vi "Message FGV.vi"(7 "Message Q FGV Actions":T2, 8 "error in":errorcluster) -> (0 "error out":errorcluster, 1 "remaining elements":T1[](array[typedef]), 2 "flushed elements":T1[](array[typedef]), 3 "queue ref out":refnum<queue>)   [LabVIEW 2020, in "Hardware.lvlib"]
doc: "Handle message queue reference operations for this component.\n\n<b>Create</b> - Obtain a message queue reference and store it in a Feedback Node.\n<b>Get</b> - Retrieve a previously stored message queue reference from the Feedback Node.\n<b>Destroy</b> - Destroy the stored message queue reference."
uses:
  Hardware.lvlib
  Message FGV Actions.ctl
  Message Type.ctl
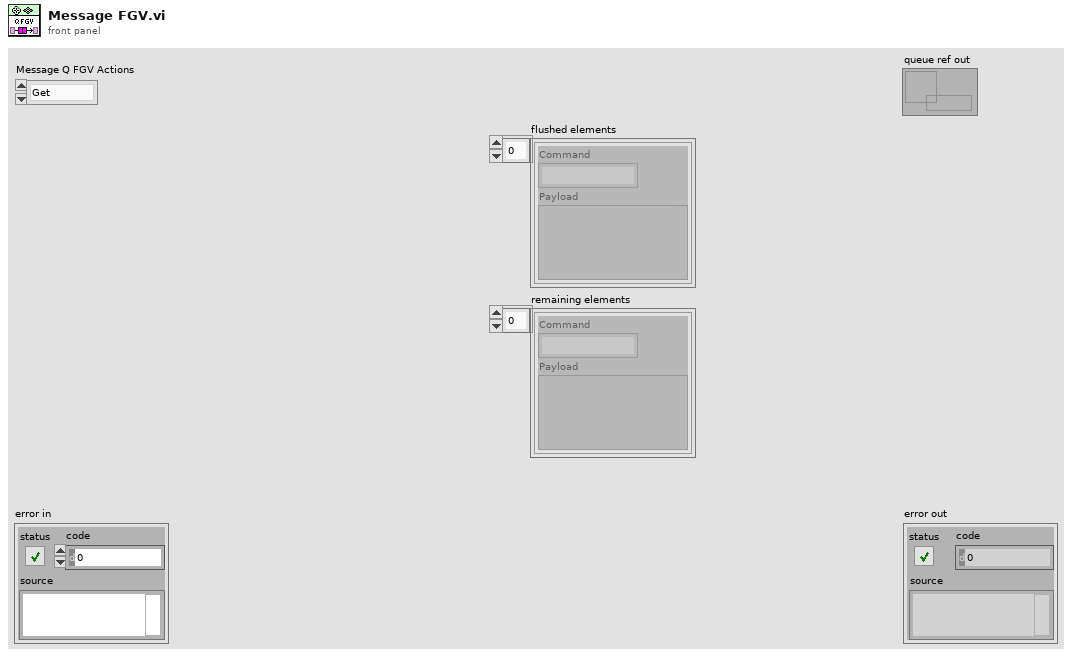
[diagram p1: front panel]
types:
  T1 = typedef "Hardware.lvlib/Message Type.ctl" = cluster{"Command":string, "Payload":variant}
  T2 = typedef "Hardware.lvlib/Message FGV Actions.ctl" = enum16{"Get", "Obtain", "Release", "Flush"}
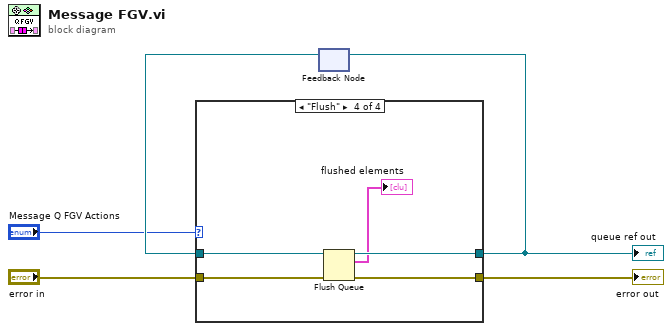
[diagram p0: block diagram]
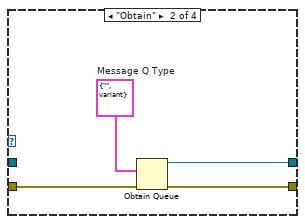
[diagram p3: hidden frame]
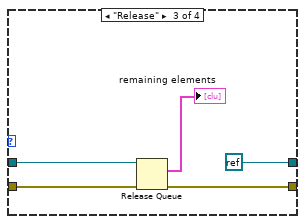
[diagram p4: hidden frame]
diagram:
  n1 = feedback #1() -> (w2:refnum<queue>)  [unwired: 1 in]
  n2 = case shown="\"Flush\"" "Message Q FGV Actions" {
    tunnel: [w6 w10 w15 w19] -> w5
    tunnel: "error in" -> [w6 w11 w16 w20]
    tunnel: [w7 w9 refnum<k0> refnum w18] -> w3
    tunnel: w2 -> [w7 _ w14 w21]
    frame "Get", Default {
    }
    frame "Obtain" {
      w8 = T1 {"Command"="", "Payload"=variant}  # Message Q Type
      n3 = Obtain Queue(element data type=w8, error in (no error)=w11) -> (queue out=w9:refnum<queue>, error out=w10:errorcluster)  [unwired: 3 in, 1 out]
    }
    frame "Release" {
      n4 = Release Queue(queue=w14, error in (no error)=w16) -> (remaining elements=→"remaining elements":T1[], error out=w15:errorcluster)  [unwired: 1 in, 1 out]
    }
    frame "Flush" {
      n5 = Flush Queue(queue=w21, error in (no error)=w20) -> (queue out=w18:refnum<queue>, remaining elements=→"flushed elements":T1[], error out=w19:errorcluster)
    }
  }
  "error out" <- w5
  "queue ref out" <- w3
  n6 = feedback-in #1(w3) -> ()
